vi "XY Scale Update.vi"(8 "error in (no error)":errorcluster, 9 "Kind":enum16{"X-Scale", "Y-Scale", "Z-Scale"}(ring), 10 "NewRange":T1, 11 "2D Plot.lvclass in":refnum<class "2D Plot.lvclass">) -> (0 "error out":errorcluster, 3 "2D Plot.lvclass out":refnum<class "2D Plot.lvclass">)   [LabVIEW 2017, in "2D Plot.lvclass"]
uses:
  <vilib>/Math Plots/2D Math Plots/2D Plot/2D Plot/2D Plot.lvclass
  <vilib>/Utility/miscctls.llb/LVRangeTypeDef.ctl
  <vilib>/Math Plots/2D Math Plots/2D Plot/2D Plot/2D Plot.lvclass/2D Plot.ctl
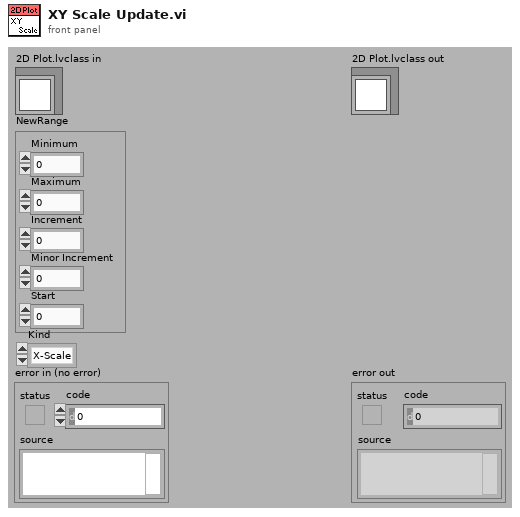
[diagram p1: front panel]
types:
  T1 = typedef "LVRangeTypeDef.ctl" = cluster{"Minimum":dbl, "Maximum":dbl, "Increment":dbl, "Minor Increment":dbl, "Start":dbl}
  T2 = typedef "2D Plot.lvclass/Scale Array.ctl" = T3[]
  T3 = typedef "2D Plot.lvclass/Scale Cluster.ctl" = cluster{"General":cluster{"Editable":bool, "Flipped":bool, "Mapping Mode":u8, "Visible":bool, "Style":u8, "Scale Fit":u8}, "Offset and Multiplier":T4, "Range":cluster{"Minimum":dbl, "Maximum":dbl, "Increment":dbl, "Minor Increment":dbl, "Start":dbl}, "Tick Color":cluster{"Major Color":u32, "Minor Color":u32}, "Gird Color":cluster{"Major Color":u32, "Minor Color":u32}, "Marker":cluster{"Visible":bool, "FG Color":u32, "BG Color":u32, "Font Name":string, "Font Size":u32, "Font Bold":bool, "Font Italic":bool, "Font Strikeout":bool, "Font Underline":bool}, "Name Label":cluster{"Visible":bool, "FG Color":u32, "BG Color":u32, "Font Name":string, "Font Size":u32, "Font Bold":bool, "Font Italic":bool, "Font Strikeout":bool, "Font Underline":bool, "Justification":enum16{"Left", "Center", "Right"}, "Text":string}}
  T4 = typedef "LVOffsetAndMultiplierTypeDef.ctl" = cluster{"Offset":dbl, "Multiplier":dbl}
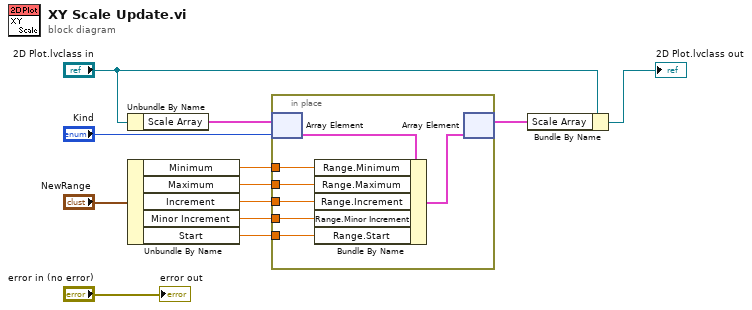
[diagram p0: block diagram]
diagram:
  n1 = Unbundle By Name("2D Plot.lvclass in") -> ("Scale Array"=w12:T2)
  n2 = Unbundle By Name("NewRange") -> ("Minimum"=w9:dbl, "Maximum"=w8:dbl, "Increment"=w7:dbl, "Minor Increment"=w6:dbl, "Start"=w5:dbl)
  n3 = in-place {
    in-place-border: w9 -> [w17]
    in-place-border: w8 -> [w16]
    in-place-border: w7 -> [w15]
    in-place-border: w6 -> [w14]
    in-place-border: w5 -> [w13]
    n4 = in-place-array #1(w12, "Kind") -> (w19:T3)
    n5 = Bundle By Name(cluster=w19, "Range.Minimum"=w17, "Range.Maximum"=w16, "Range.Increment"=w15, "Range.Minor Increment"=w14, "Range.Start"=w13) -> (w18:T3)
    n6 = in-place-array #1(w18) -> (w4:T2)  [unwired: 1 out]
  }
  n7 = Bundle By Name(cluster="2D Plot.lvclass in", "Scale Array"=w4) -> (→"2D Plot.lvclass out":refnum<class "2D Plot.lvclass">)
  "error out" <- "error in (no error)"
